vi "draw vert line.vi"(11 "Refnum in":T1) -> (3 "Refnum out":T1)   [LabVIEW 2015]
uses:
  <vilib>/vision/Image Controls.llb/IMAQ Image.ctl
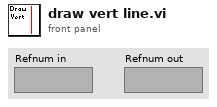
[diagram p1: front panel]
types:
  T1 = typedef "IMAQ Image.ctl" = refnum<image>
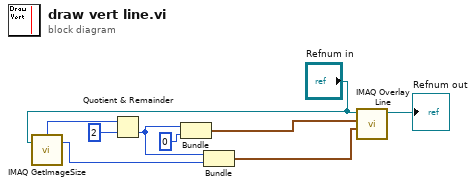
[diagram p0: block diagram]
diagram:
  n1 = call "IMAQ GetImageSize"("Image"="Refnum in") -> ("Y Resolution"=w8:i32, "X Resolution"=w2:i32)  [unwired: 3 in, 1 out]
  n2 = Quotient & Remainder(x=w2, y=2) -> (floor(x/y)=w5:i32)  [unwired: 1 out]
  n3 = Bundle(w5, "y"=0) -> (w4:cluster{i32, "y":i32})  [unwired: 1 in]
  n4 = Bundle(w5, "Y Resolution"=w8) -> (w6:cluster{i32, "Y Resolution":i32})  [unwired: 1 in]
  n5 = call "IMAQ Overlay Line"("End Point"=w6, "Start Point"=w4, "Image"="Refnum in") -> ("Image Out"=→"Refnum out":T1)  [unwired: 7 in, 1 out]
